vi "Compare Seq Numbers.vi"(8 "B":u16, 11 "A":u16) -> (0 "A Greater Than B":bool, 3 "A equals B":bool)   [LabVIEW 2017]
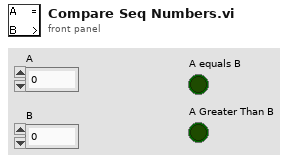
[diagram p1: front panel]
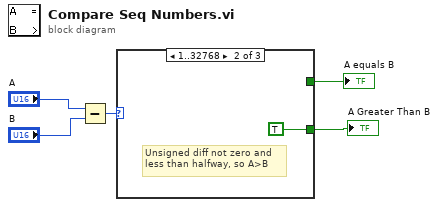
[diagram p0: block diagram]
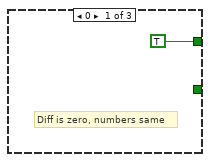
[diagram p2: hidden frame]
diagram:
  n1 = Subtract(x="A", y="B") -> (x-y=w3:u16)
  n2 = case shown="1..32768" w3 {
    tunnel: [TRUE _ _] -> w2
    tunnel: [_ TRUE _] -> w1
    frame 0 {
      # "Diff is zero, numbers same"
    }
    frame 1..32768 {
      # "Unsigned diff not zero and\nless than halfway, so A>B"
    }
    frame Default {
      # "B>A"
    }
  }
  "A equals B" <- w2
  "A Greater Than B" <- w1
